vi "space.vi"() -> (3 "_":u8)   [LabVIEW 2025, in "AOC.lvlib"]
uses:
  AOC.lvlib
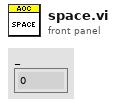
[diagram p1: front panel]
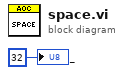
[diagram p0: block diagram]
diagram:
  "_" <- u8 32 ("element")
